vi "Update Message.vi"(8 "error in (no error)":errorcluster, 10 "Sequence Context In":refnum<k7>, 11 "TestExec in":refnum<class "TestExec.lvclass">) -> (0 "error out":errorcluster, 3 "TestExec out":refnum<class "TestExec.lvclass">)   [LabVIEW 2019, in "Sequence Main.lvlib" / "TestExec.lvclass"]
uses:
  TestExec.lvclass
  TestExec.lvclass/TestExec.ctl
  cf93842d-14b4-48e3-8168-b31a3e48433b.vi
  <vilib>/addons/TestStand/_TSUtility.llb/TestStand - Get Property Value (String).vi
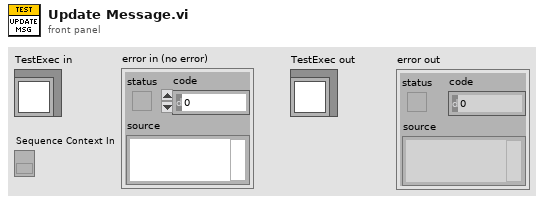
[diagram p1: front panel]
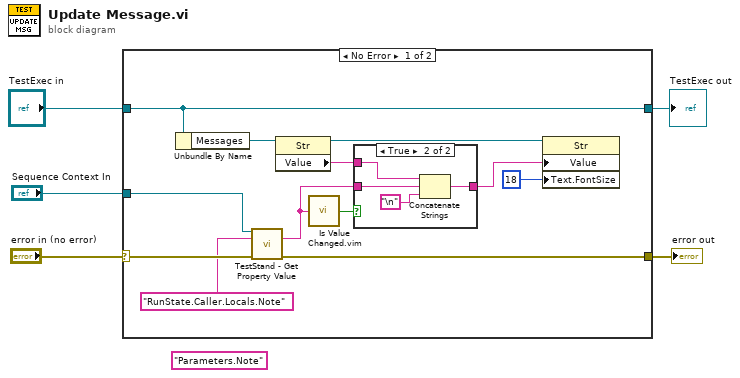
[diagram p0: block diagram]
diagram:
  (unwired) "Parameters.Note" ("Lookup String")
  n1 = case shown="No Error" "error in (no error)" {
    selector: "error in (no error)" -> [w17 w24]
    tunnel: [w11 w24] -> w4
    tunnel: [w16 w23] -> w2
    tunnel: "TestExec in" -> [w16 w23]
    tunnel: "Sequence Context In" -> [w10 _]
    frame No Error {
      n2 = Unbundle By Name(w16) -> ("Messages"=w13:refnum<vi>)
      n3 = call-poly <vilib>:"TestStand - Get Property Value.vi"("Sequence Context In"=w10, "Lookup String"="RunState.Caller.Locals.Note", "error in (no error)"=w17) -> ("Value"=w6:string, "error out"=w11:errorcluster)  [unwired: 10 in, 1 out]
      n4 = property class="Str"(reference=w13) -> (reference out=w12:refnum<vi>, "Value"=w14:string)  [unwired: 1 in, 1 out]
      n5 = call "Is Value Changed.vim"("value"=w6) -> ("changed or first call?"=w7:bool)
      n6 = case shown="True" w7 {
        tunnel: w14 -> [w18 w22]
        tunnel: [w18 w21] -> w8
        tunnel: w6 -> [_ w20]
        frame False {
        }
        frame True {
          n7 = Concatenate Strings(w22, w20, "\n") -> (w21:string)
        }
      }
      n8 = property class="Str"(reference=w12, "Value"=w8, "Text.FontSize"=u32 18 ("Text.Font:Size")) -> ()  [unwired: 1 in, 2 out]
    }
    frame Error {
    }
  }
  "error out" <- w4
  "TestExec out" <- w2
